vi "ma_Two-sided FFT Spectrum (CDB).vi"(8 "error in":errorcluster, 10 "dt":dbl format="%0.2f", 11 "signal (V)":cdb[](array[numeric]) format="%0.2f") -> (0 "error out":errorcluster, 1 "f0":dbl format="%0.2f", 2 "df":dbl format="%0.2f", 3 "FFT spectrum (Vrms)":cdb[](array[numeric]) format="%0.2f")   [LabVIEW 2020, in "NI_MAPro.lvlib"]
uses:
  NI_MAPro.lvlib
  NI_AALPro.lvlib
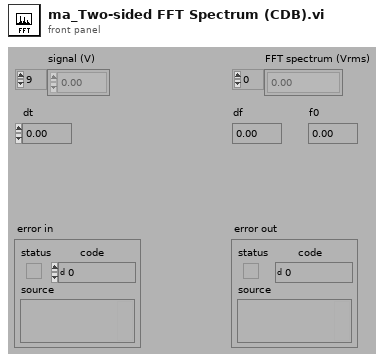
[diagram p1: front panel]
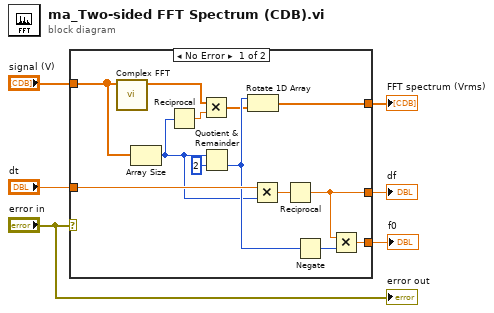
[diagram p0: block diagram]
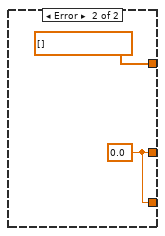
[diagram p2: hidden frame]
diagram:
  n1 = case shown="No Error" "error in" {
    tunnel: "signal (V)" -> [w18 _]
    tunnel: [w17 cdb[] [] ("one-sided spectrum (complex)")] -> w5
    tunnel: "dt" -> [w19 _]
    tunnel: [w14 w20] -> w3
    tunnel: [w11 w20] -> w1
    frame No Error {
      n2 = call "Complex FFT.vi"("X"=w18) -> ("FFT {X}"=w8:cdb[])  [unwired: 9 in, 1 out]
      n3 = Array Size(array=w18) -> (size(s)=w10:i32)
      n4 = Reciprocal(x=w10) -> (1/x=w9:dbl)
      n5 = Multiply(x=w8, y=w9) -> (x*y=w7:cdb[])
      n6 = Quotient & Remainder(x=w10, y=2) -> (floor(x/y)=w13:i32)  [unwired: 1 out]
      n7 = Rotate 1D Array(1:w7, 2:w13) -> (0:w17:cdb[])
      n8 = Multiply(x=w19, y=w10) -> (x*y=w15:dbl)
      n9 = Reciprocal(x=w15) -> (1/x=w14:dbl)
      n10 = Negate(x=w13) -> (-x=w12:i32)
      n11 = Multiply(x=w14, y=w12) -> (x*y=w11:dbl)
    }
    frame Error {
      w20 = 0.0
    }
  }
  "df" <- w3
  "FFT spectrum (Vrms)" <- w5
  "f0" <- w1
  "error out" <- "error in"
